vi "COMTRADE Read Private Inf.vi"   [LabVIEW 2012, in "NI_EP_COMTRADE.lvlib"]
doc: "Reads information from the private sections of the optionally specified .inf file. You must set <B>open mode</B> to Open (read only) in the COMTRADE Open VI to open the .inf file. Otherwise this VI returns an error."
uses:
  <vilib>/addons/Electrical Power/File IO/NI_EP_COMTRADE.lvlib
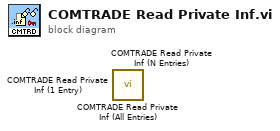
[diagram p0: block diagram]
diagram:
  n1 = call <vilib>:"COMTRADE Read Private Inf (All Entries).vi"() -> ()  [unwired: 8 in, 4 out]
  n2 = call <vilib>:"COMTRADE Read Private Inf (N Entries).vi"() -> ()  [unwired: 8 in, 4 out]
  n3 = call <vilib>:"COMTRADE Read Private Inf (1 Entry).vi"() -> ()  [unwired: 8 in, 4 out]
